vi "stop_can_master.vi"() -> (3 "return":i16)   [LabVIEW 2011]
uses:
  canopen_dll_master.dll
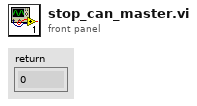
[diagram p1: front panel]
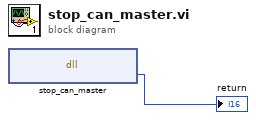
[diagram p0: block diagram]
diagram:
  n1 = dll-call lib="canopen_dll_master.dll" fn="stop_can_master"() -> ("return type"=→"return":i16)  [unwired: 3 in, 2 out]
